vi "MEE5318_Project2_Walker_Duffy.vi"() -> ()   [LabVIEW 2021]
doc: "I. Description:\nThis example demonstrates how to continuously acquire and generate data at the same time, synchronized with one another.\n\nII. Instructions for Running:\n1. Select the physical channel to correspond to where your signal is input on the DAQ device. Also, select the corresponding channel for where your signal is being generated.\n2. Enter the minimum and maximum voltage ranges.\nNote: For better accuracy try to match the input range to the expected voltage level of the measured signal.\n3. Set the sample rate of the acquisition.\nNote: The rate should be at least twice as fast as the maximum frequency component of the signal being acquired. \n6. Select the Rate for the generation\n7. Select what type of signal to generate and the amplitude.\nNote: This example requires two DMA channels to run. If your hardware does not support two DMA channels, you need to set the Data Transfer Mechanism property for the Analog Output Task to use \"Interrupts\". The Data Transfer Mechanism property is located in the DAQmx Channel Property hierarchy at:\n\nDAQmx Channel Property Node>>Analog Output>>General Properties>>Advanced>>Data Transfer and Memory>>Data Transfer Mechanism\n\nRefer to your device documentation to determine how many DMA channels are supported for your hardware.\n\nIII. Block Diagram Steps:\n1. Create an analog input voltage channel. Also, create an analog output voltage channel.\n2. Set the rate for the sample clock. Additionally, define the sample mode to be continuous. Also, set the sample clock rate for the signal generation.\n2a. Call the Get Terminal Name with Device Prefix VI. This will take a Task and a terminal and create a properly formatted device + terminal name to use as the source of the Trigger.\n3. Define the parameters for a Digital Edge Start Trigger. Set the Analog output to trigger off the AI Start Trigger. This is an internal trigger signal.\n4. Use the Basic Function Generator VI to create the signal to be generated.\n5. Call the Start VI to arm the two functions. Make sure the analog output is armed before the analog input. This will ensure both will start at the same time.\n6. Read the waveform data in a loop until the user hits the stop button or an error occurs. The Is Task Done? VI is used to check for errors in the Analog Output Task.\n7. Call the Clear VI to Clear the Task\n8. Use the popup dialog box to display an error if any.\n\nIV. I/O Connections Overview:\nMake sure your signal input/output terminals match the Physical Channel I/O controls."
uses:
  <vilib>/DAQmx/write.llb/DAQmx Write (Analog Wfm 1Chan NSamp).vi
  <vilib>/DAQmx/read.llb/DAQmx Read (Analog 1D Wfm NChan NSamp).vi
  <vilib>/DAQmx/create/channels.llb/DAQmx Create Channel (AI-Voltage-Basic).vi
  <vilib>/DAQmx/create/channels.llb/DAQmx Create Channel (AO-Voltage-Basic).vi
  <vilib>/DAQmx/configure/timing.llb/DAQmx Timing (Sample Clock).vi
  <vilib>/Utility/file.llb/Write Delimited Spreadsheet (string).vi
  <vilib>/DAQmx/miscellaneous.llb/DAQmx Fill In Error Info.vi
  <vilib>/measure/maspectr.llb/FFT Spectrum (Mag-Phase) for 1 Chan.vi
  <vilib>/measure/matone.llb/Extract Single Tone Information 1 Chan.vi
  <vilib>/Utility/file.llb/Write Delimited Spreadsheet (DBL).vi
  <resource>/objmgr/daqmx.rc
  <vilib>/measure/NI_MAPro.lvlib
  <vilib>/measure/NI_MABase.lvlib
panel:
  out "XY Graph 6":cluster{dbl[], dbl[]}(graph)={[1.003442506962999, 1.2610992094523745, 1.5837726092934932, 1.995784074596131, 2.511945155284467, 3.162284743422122, 3.981122144935631, 5.01179955506919, 6.309703700351375, 7.943258071381784, 10.000055566779254, 12.58939934275368, 15.84904372029721, 19.952629650432385, 25.11898815046962, 31.622975651338173, 39.810782329385304, 50.11908125109304, 63.09615289925839, 79.4332134036227, 100.00056628183589, 125.89213042712618, 158.48949946329975, 199.52632880375762, 251.1892045181882, 316.22825265681826, 398.1077651482482, 501.18772990572995, 630.9567660427073, 794.3285341092678, 1000.0006588922621, 1258.924838656023, 1584.8926393467586, 1995.26271005492, 2511.8858646104495, 3162.2780352316154, 3981.0723110331146, 5011.871748610918, 6309.573284192407, 7943.282718567373, 10000.00070613037, 12589.254486271182, 15848.931335861447, 19952.622951606714, 25118.863844313797], [4.705942162303998, 4.904408419943991, 4.500687842745691, 4.406572166079357, 8.904479438365001, 10.965330019855998, 13.31846259250105, 15.897946390893196, 18.475090576808327, 20.80876079957578, 22.561101244931443, 23.403589846634034, 23.180444668855472, 21.983239153585146, 20.02387193704839, 17.60063463697611, 15.046945360814675, 12.583523146700912, 10.338346218640638, 8.345289183655666, 6.607581916375594, 5.082440939814717, 3.754990748114679, 2.5419716823078105, 1.4053842328342512, 0.2903218305122266, -0.8625405477539232, -2.1065937127375918, -3.5185386397777734, -5.137086709227759, -7.057912744275114, -9.358439054857229, -12.12461093428385, -15.434887120432961, -19.33029359124265, -23.795887799181287, -28.69190886134045, -33.69336120946643, -38.302524962207144, -41.88419344064653, -44.00034802863394, -43.50651100659074, -40.77568318478461, -35.56439084500755, -28.078585789859645]}
  out "XY Graph 5":cluster{dbl[], dbl[]}(graph)={[1.0011090357381531, 1.2591626691701139, 1.5846117134075075, 1.9953177308690426, 2.5119207737576486, 3.1622929612779918, 3.9810907133666693, 5.01184827533032, 6.309660904978634, 7.943241093294676, 10.00007090370485, 12.589397101066721, 15.84897313183063, 19.952605454788852, 25.119030529667754, 31.6229724447658, 39.81077296749638, 50.119081095454064, 63.09617380683147, 79.43323069559837, 100.00057222422406, 125.89213381652905, 158.48951312715062, 199.52632988171456, 251.18919438848772, 316.2282504086257, 398.1077638655443, 501.18774701521585, 630.9567526678833, 794.3285331758716, 1000.0006686882722, 1258.9248376169114, 1584.892637256621, 1995.262708195959, 2511.8858710728996, 3162.278037210249, 3981.0722988514854, 5011.871748537684, 6309.573310573001, 7943.282691591783, 9999.99932913371, 12589.254476409284, 15848.931339797815, 19952.62294183974, 25118.863785275887], [-22.295857945666143, -22.25349261876203, -22.195324800268807, -22.13801141426177, -22.04049018857964, -21.891483667442422, -21.66880706135075, -21.34849578708461, -20.908928022499094, -20.339831588390208, -19.652903791038298, -18.886274774838473, -18.102460970662406, -17.363632344083346, -16.722607777856634, -16.201761703016857, -15.803079135588538, -15.510034326649837, -15.30025445676455, -15.15183614910715, -15.048501486636248, -14.978006333004945, -14.926598238261606, -14.889246997153315, -14.860801987931126, -14.839403891060956, -14.824153226115737, -14.816139312238555, -14.8164519690332, -14.829306612388514, -14.860428961170593, -14.919199872906203, -15.021259960399453, -15.190264519268336, -15.456771957684163, -15.865631434255699, -16.46459308249321, -17.306129381000332, -18.428054521729482, -19.838845372404887, -21.508587770236346, -23.38690486265571, -25.406404731582132, -27.515566437722537, -29.684106370075064]}
  out "Gain Plot 6":cluster{"f0":dbl, "df":dbl, dbl[]}(graph)={"f0"=0.0, "df"=1.0, array[50000 elements]} caption="Gain"
  in  "Samples per Decade":dbl=10.0
  in  "ending frequency":dbl=20000.0 format="%0.2p"
  in  "file path":path=path "E:/School/FIT/Spring 2022/MEE 5318/Project #2/data.csv"
  in  "starting frequency":dbl=1.0 format="%0.2p"
  out "Time Domain":waveform(dbl)[](graph)=[{"t0"=timestamp(3733250361.6547537 s since 1904-01-01), "dt"=9.999999999999972e-06, "Y"=array[100000 elements], "attributes"=variant("NI_ChannelName"=variant(string "myDAQ1/ai0"), "NI_UnitDescription"=variant(string "Volts"))}, {"t0"=timestamp(3733250361.654759 s since 1904-01-01), "dt"=9.999999999999972e-06, "Y"=array[100000 elements], "attributes"=variant("NI_ChannelName"=variant(string "myDAQ1/ai1"), "NI_UnitDescription"=variant(string "Volts"))}]
  in  "Sampling Info":T1={"Sampling Rate"=100000.0, "Number of Samples per loop"=100000} {"Sampling Rate" format="%.2p"}
  in  "Amplitude":dbl=1.0 format="%0.2p"
  in  "Channel":tag="myDAQ1/ao0" caption="Output Physical Channels"
  in  "Channel":tag="myDAQ1/ai0:1" caption="Input Physical Channel"
  # "Channel Parameters"
  # "Signal Generation"
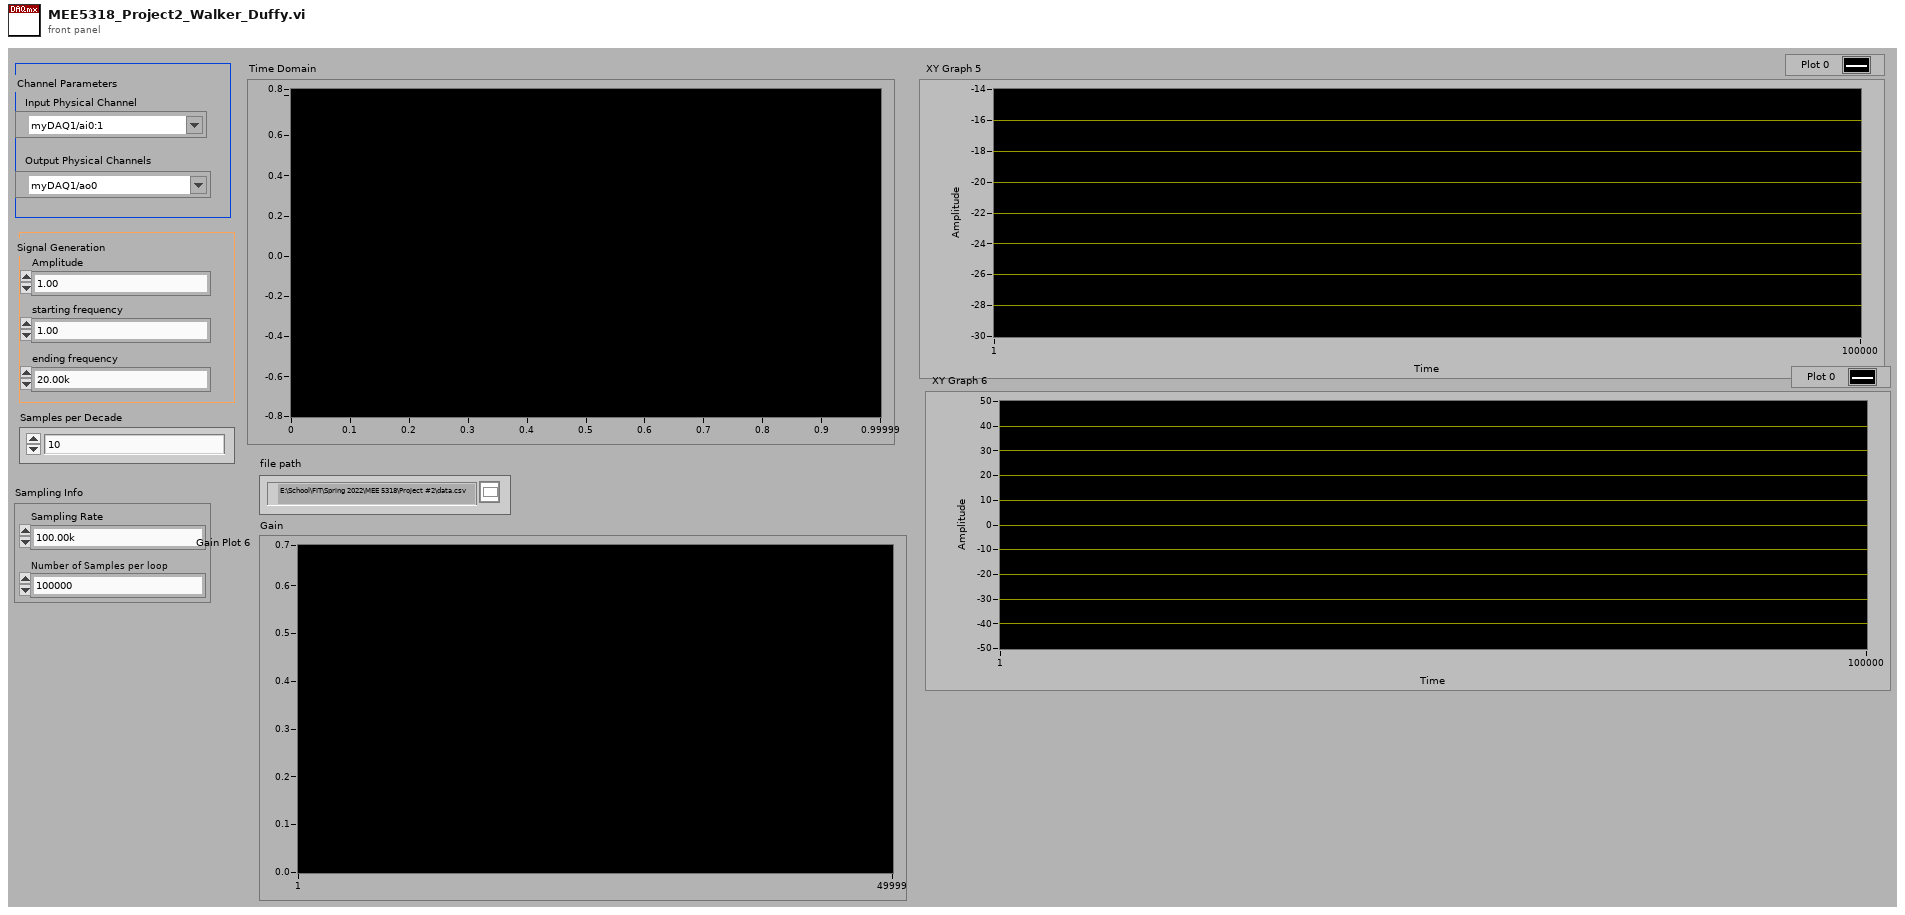
[diagram p1: front panel]
types:
  T1 = cluster{"Sampling Rate":dbl, "Number of Samples per loop":u32}
  T2 = enum32{"none", "input signal", "detected signal", "residual signal"}
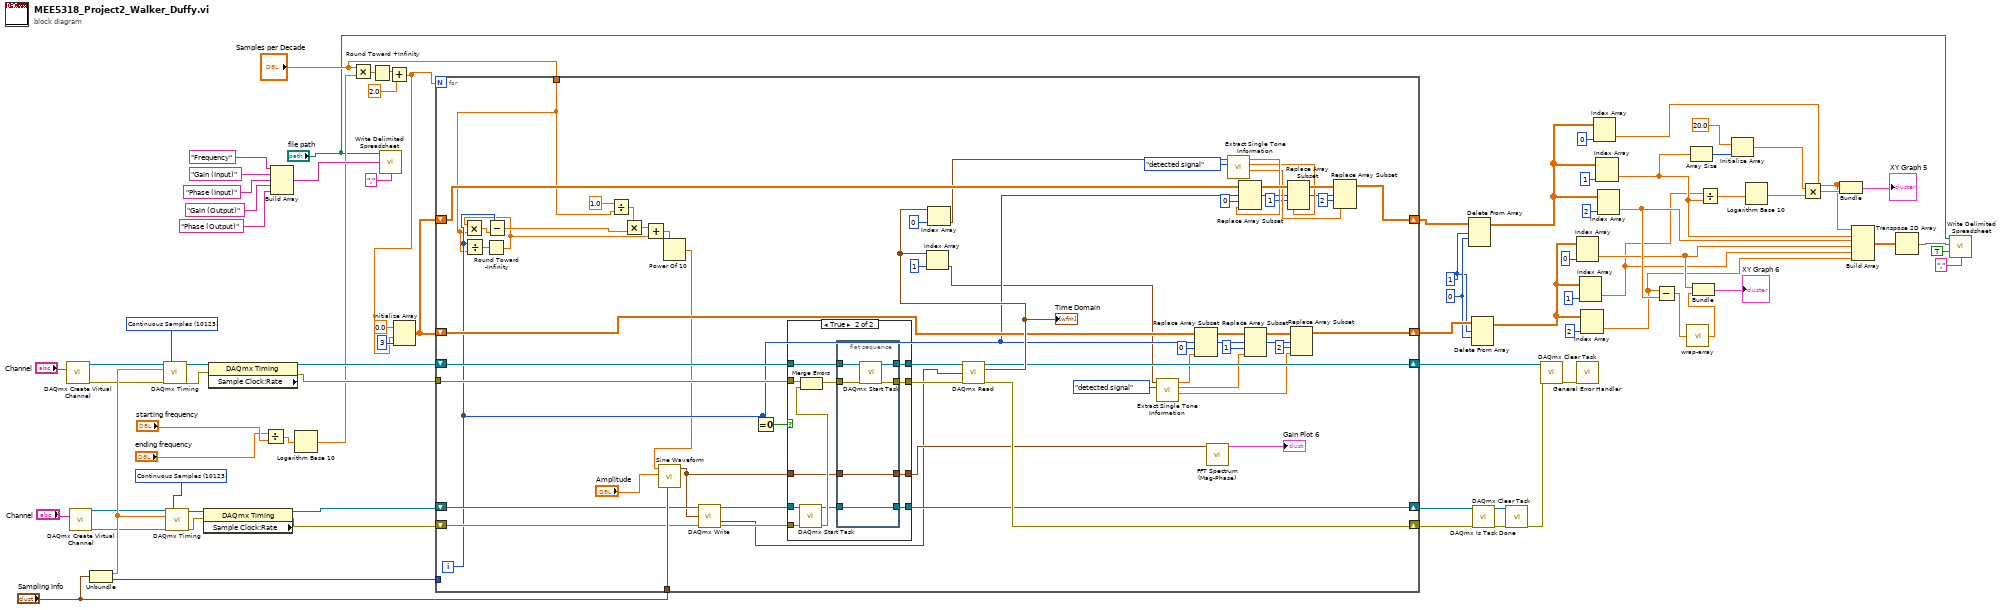
[diagram p0: block diagram]
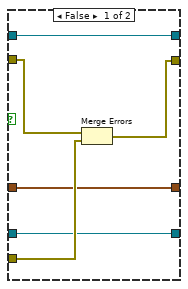
[diagram p2: hidden frame]
diagram:
  w25 = 1 ("length")
  w26 = 0 ("index (row)")
  w54 = 10123 items=["Finite Samples"=10178, "Continuous Samples"=10123] ("sample mode")
  w61 = 10123 items=["Finite Samples"=10178, "Continuous Samples"=10123] ("sample mode")
  n1 = call-poly <vilib>:"DAQmx Create Virtual Channel.vi"("physical channels"="Channel") -> ("task out"=w63:refnum<k21>, "error out"=w62:errorcluster)  [unwired: 13 in]
  n2 = call-poly <vilib>:"DAQmx Create Virtual Channel.vi"("physical channels"="Channel") -> ("task out"=w65:refnum<k21>, "error out"=w66:errorcluster)  [unwired: 13 in]
  n3 = Unbundle("Sampling Info") -> ("Sampling Rate"=w78:dbl, "Number of Samples per loop"=w20:u32)
  n4 = call-poly <vilib>:"DAQmx Timing.vi"("task/channels in"=w63, "sample mode"=w61, "rate"=w78, "error in"=w62) -> ("task out"=w72:refnum<k21>, "error out"=w73:errorcluster)  [unwired: 10 in]
  n5 = call-poly <vilib>:"DAQmx Timing.vi"("task/channels in"=w65, "sample mode"=w54, "rate"=w78, "error in"=w66) -> ("task out"=w70:refnum<k21>, "error out"=w71:errorcluster)  [unwired: 10 in]
  n6 = property class="DAQmx Timing" props=["Sample Clock:Rate"](reference=w70, error in=w71) -> (reference out=w57:refnum<k21>, error out=w56:errorcluster)  [unwired: 1 out]
  n7 = property class="DAQmx Timing" props=["Sample Clock:Rate"](reference=w72, error in=w73) -> (reference out=w59:refnum<k21>, error out=w58:errorcluster)  [unwired: 1 out]
  n8 = Divide(x="ending frequency", y="starting frequency") -> (x/y=w24:dbl)
  n9 = Build Array("Frequency", "Gain (Input)", "Phase (Input)", "Gain (Output)", "Phase (Output)") -> (w52:string[])
  n10 = Logarithm Base 10(1:w24) -> (0:w19:dbl)
  n11 = Multiply(x="Samples per Decade", y=w19) -> (x*y=w18:dbl)
  n12 = Round Toward +Infinity(x=w18) -> (ceil(x): smallest int >= x=w5:dbl)
  n13 = call-poly <vilib>:"Write Delimited Spreadsheet.vi"("file path (dialog if empty)"="file path", "1D data"=w52, "delimiter (\\t)"="," ("delimiter (\\t)")) -> ()  [unwired: 11 in, 2 out]
  n14 = Add(x=w5, y=2.0) -> (x+y=w6:dbl)
  n15 = Initialize Array(0.0 ("element"), w6, 3 ("dimension size")) -> (w46:dbl[][])
  n16 = for {
    N: w6 -> [_]
    tunnel: "Sampling Info" -> [w134]
    tunnel: w58 -> [w124]
    shift-right: [w122] -> w67
    shift-left: w57 -> [w131]
    shift-right: [w123] -> w77
    shift-left: w56 -> [w130]
    shift-right: [w118] -> w60
    shift-left: w59 -> [w125]
    shift-right: [w110] -> w28
    shift-left: w46 -> [w116]
    shift-right: [w98] -> w30
    shift-left: w46 -> [w97]
    tunnel: "Samples per Decade" -> [w84]
    tunnel: w20 -> [_]
    i -> [w91]
    n17 = Divide(x=w91, y=w84) -> (x/y=w93:dbl)
    n18 = Round Toward -Infinity(1:w93) -> (0:w79:dbl)
    n19 = Multiply(x=w79, y=w84) -> (x*y=w92:dbl)
    n20 = Subtract(x=w91, y=w92) -> (x-y=w81:dbl)
    n21 = Divide(x=1.0, y=w84) -> (x/y=w83:dbl)
    n22 = Multiply(x=w83, y=w81) -> (x*y=w82:dbl)
    n23 = Add(x=w82, y=w79) -> (x+y=w80:dbl)
    n24 = Power Of 10(x=w80) -> (10^x=w86:dbl)
    n25 = call <vilib>:"Sine Waveform.vi"("sampling info"=w134, "amplitude"="Amplitude", "frequency"=w86) -> ("signal out"=w94:waveform(dbl))  [unwired: 7 in, 1 out]
    n26 = call-poly <vilib>:"DAQmx Write.vi"("task/channels in"=w131, "data"=w94, "error in"=w130) -> ("task out"=w128:refnum<k21>, "number of samples written per channel"=w87:u32, "error out"=w129:errorcluster)  [unwired: 10 in]
    n27 = Equal To 0?(x=w91) -> (x = 0?=w121:bool)
    n28 = case shown="True" w121 {
      tunnel: [w138 w152] -> w133
      tunnel: [w137 w149] -> w132
      tunnel: w129 -> [w140 w148]
      tunnel: w128 -> [w136 w147]
      tunnel: w125 -> [w137 w146]
      tunnel: w124 -> [w139 w145]
      tunnel: [w136 w143] -> w122
      tunnel: w94 -> [w135 w142]
      tunnel: [w135 w141] -> w95
      frame False {
        n29 = Merge Errors(w139, w140) -> (w138:errorcluster)
      }
      frame True {
        n30 = call <vilib>:"DAQmx Start Task.vi"("task/channels in"=w147, "error in"=w148) -> ("task out"=w144:refnum<k21>, "error out"=w150:errorcluster)  [unwired: 12 in]
        n31 = Merge Errors(w145, w150) -> (w151:errorcluster)
        n32 = flat-sequence {
          tunnel: [w158] -> w152
          tunnel: w151 -> [w157]
          tunnel: [w156] -> w149
          tunnel: w146 -> [w155]
          tunnel: w144 -> [w154]
          tunnel: [w154] -> w143
          tunnel: w142 -> [w153]
          tunnel: [w153] -> w141
          frame #0 {
            n33 = call <vilib>:"DAQmx Start Task.vi"("task/channels in"=w155, "error in"=w157) -> ("task out"=w156:refnum<k21>, "error out"=w158:errorcluster)  [unwired: 12 in]
          }
        }
      }
    }
    n34 = call-poly <vilib>:"DAQmx Read.vi"("task/channels in"=w132, "number of samples per channel"=w87, "error in"=w133) -> ("task out"=w118:refnum<k21>, "data"=w120:waveform(dbl)[], "error out"=w123:errorcluster)  [unwired: 10 in]
    "Time Domain" <- w120
    n35 = Index Array(array=w120, index=1) -> (element=w89:waveform(dbl))
    n36 = Index Array(array=w120, index=0) -> (element=w88:waveform(dbl))
    n37 = call-poly <vilib>:"Extract Single Tone Information.vi"("export mode"=T2."detected signal", "time signal in"=w89) -> ("detected phase (deg)"=w108:dbl, "detected amplitude"=w113:dbl, "detected frequency"=w112:dbl)  [unwired: 4 in, 3 out]
    n38 = Replace Array Subset(array=w116, new element=w112, index (row)=w91, index (col)=0 ("disabled index (col)")) -> (w117:dbl[][])
    n39 = call-poly <vilib>:"FFT Spectrum (Mag-Phase).vi"("time signal"=w95) -> ("magnitude"=→"Gain Plot 6":cluster{"f0":dbl, "df":dbl, "magnitude":dbl[]})  [unwired: 6 in, 4 out]
    n40 = call-poly <vilib>:"Extract Single Tone Information.vi"("export mode"=T2."detected signal", "time signal in"=w88) -> ("detected phase (deg)"=w99:dbl, "detected amplitude"=w100:dbl, "detected frequency"=w101:dbl)  [unwired: 4 in, 3 out]
    n41 = Replace Array Subset(array=w97, new element=w101, index (row)=w91, index (col)=0 ("disabled index (col)")) -> (w105:dbl[][])
    n42 = Replace Array Subset(array=w117, new element=w113, index (row)=w91, index (col)=1 ("disabled index (col)")) -> (w111:dbl[][])
    n43 = Replace Array Subset(array=w105, new element=w100, index (row)=w91, index (col)=1 ("disabled index (col)")) -> (w103:dbl[][])
    n44 = Replace Array Subset(array=w111, new element=w108, index (row)=w91, index (col)=2 ("disabled index (col)")) -> (w110:dbl[][])
    n45 = Replace Array Subset(array=w103, new element=w99, index (row)=w91, index (col)=2 ("disabled index (col)")) -> (w98:dbl[][])
  }
  n46 = Delete From Array(array=w30, length=w25, index (row)=w26) -> (array with subset deleted=w29:dbl[][])  [unwired: 1 in, 1 out]
  n47 = Delete From Array(array=w28, length=w25, index (row)=w26) -> (array with subset deleted=w27:dbl[][])  [unwired: 1 in, 1 out]
  n48 = call <vilib>:"DAQmx Is Task Done.vi"("task/channels in"=w67, "error in"=w77) -> ("task out"=w68:refnum<k21>, "error out"=w74:errorcluster)  [unwired: 11 in, 1 out]
  n49 = call <vilib>:"DAQmx Clear Task.vi"("task in"=w68, "error in"=w74) -> ("error out"=w75:errorcluster)  [unwired: 13 in]
  n50 = call <vilib>:"DAQmx Clear Task.vi"("task in"=w60, "error in"=w75) -> ("error out"=w76:errorcluster)  [unwired: 13 in]
  n51 = Index Array(array=w27, index (col)=0 ("disabled index (col)")) -> (element=w10:dbl[])  [unwired: 1 in]
  n52 = call <vilib>:"General Error Handler.vi"("error in (no error)"=w76) -> ()  [unwired: 10 in, 5 out]
  n53 = Index Array(array=w27, index (col)=1 ("disabled index (col)")) -> (element=w9:dbl[])  [unwired: 1 in]
  n54 = Index Array(array=w27, index (col)=2 ("disabled index (col)")) -> (element=w8:dbl[])  [unwired: 1 in]
  n55 = Index Array(array=w29, index (col)=0 ("disabled index (col)")) -> (element=w11:dbl[])  [unwired: 1 in]
  n56 = Index Array(array=w29, index (col)=1 ("disabled index (col)")) -> (element=w12:dbl[])  [unwired: 1 in]
  n57 = Index Array(array=w29, index (col)=2 ("disabled index (col)")) -> (element=w13:dbl[])  [unwired: 1 in]
  n58 = Subtract(x=w8, y=w13) -> (x-y=w2:dbl[])
  n59 = call "wrap-array.vi"("Array In"=w2) -> ("Array Out"=w1:dbl[])
  n60 = Array Size(array=w12) -> (size(s)=w40:i32)
  n61 = Bundle(w10, "Array Out"=w1) -> (→"XY Graph 6":cluster{dbl[], "Array Out":dbl[]})  [unwired: 1 in]
  n62 = Divide(x=w9, y=w12) -> (x/y=w41:dbl[])
  n63 = Initialize Array(20.0 ("element"), w40) -> (w38:dbl[])
  n64 = Logarithm Base 10(1:w41) -> (0:w42:dbl[])
  n65 = Multiply(x=w38, y=w42) -> (x*y=w36:dbl[])
  n66 = Bundle(w11, w36) -> (→"XY Graph 5":cluster{dbl[], dbl[]})  [unwired: 1 in]
  n67 = Build Array(w11, w12, w13, w10, w9, w8) -> (w17:dbl[][])
  n68 = Transpose 2D Array(2D array=w17) -> (transposed array=w14:dbl[][])
  n69 = call-poly <vilib>:"Write Delimited Spreadsheet.vi"("file path (dialog if empty)"="file path", "2D data"=w14, "append to file? (new file:F)"=TRUE, "delimiter (\\t)"="," ("delimiter (\\t)")) -> ()  [unwired: 10 in, 2 out]
